vi "GetProperties.vi"(8 "error in":errorcluster, 11 "Numeric in":refnum<class "Numeric.lvclass">) -> (0 "error out":errorcluster, 3 "Numeric out":refnum<class "Numeric.lvclass">)   [LabVIEW 2014, in "Numeric.lvclass"]
uses:
  Numeric.lvclass
  Numeric.lvclass/Numeric.ctl
  Control/Control.lvclass
  Text/Text.lvclass
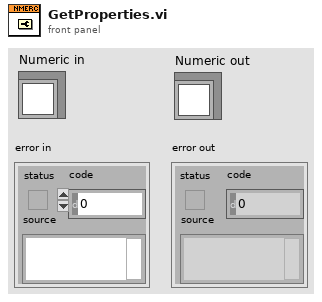
[diagram p1: front panel]
types:
  T1 = typedef "LVMinMaxIncTypeDef.ctl" = cluster{"Minimum":dbl, "Maximum":dbl, "Increment":dbl}
  T2 = typedef "LVKeyTypeDef.ctl" = cluster{"Focus":bool, "Control":bool, "Shift":bool, "Key":string}
  T3 = typedef "LVNumericRepresentation.ctl" = enum32{"Extended Precision", "Double Precision", "Single Precision", "Long", "Word", "Byte", "Unsigned Long", "Unsigned Word", "Unsigned Byte", "Complex Extended", "Complex Double", "Complex Single", "Quad", "Unsigned Quad", "Fixed-Point"}
  T4 = typedef "LVOutOfRangeActionTypeDef.ctl" = cluster{"OutOfRngActMin":u8, "OutOfRngActMax":u8, "OutOfRngActInc":u8}
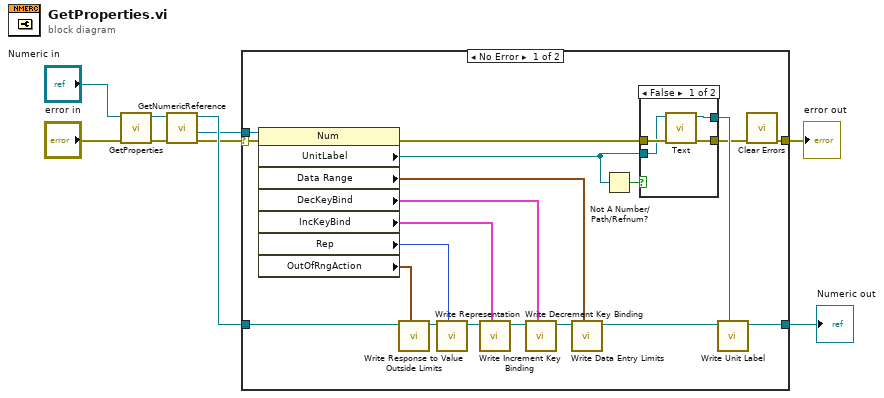
[diagram p0: block diagram]
diagram:
  n1 = call-parent "GetProperties.vi"("error in"="error in", "Control in"="Numeric in") -> ("error out"=w1:errorcluster, "Control out"=w4:refnum<class "Numeric.lvclass">)  [unwired: 8 in]
  n2 = call "GetNumericReference.vi"("error in"=w1, "Numeric in"=w4) -> ("error out"=w6:errorcluster, "Numeric reference"=w5:refnum<vi>, "Numeric out"=w7:refnum<class "Numeric.lvclass">)  [unwired: 7 in]
  n3 = case shown="No Error" w6 {
    selector: w6 -> [w29 w36]
    tunnel: [w10 w36] -> w9
    tunnel: [w12 w35] -> w8
    tunnel: w5 -> [w28 _]
    tunnel: w7 -> [w13 w35]
    frame No Error {
      n4 = property class="Num"(reference=w28, error in=w29) -> (error out=w27:errorcluster, "UnitLabel"=w25:refnum<vi>, "Data Range"=w17:T1, "DecKeyBind"=w18:T2, "IncKeyBind"=w19:T2, "Rep"=w22:T3, "OutOfRngAction"=w23:T4)  [unwired: 1 out]
      n5 = call "Write Response to Value Outside Limits.vi"("Out of Range Action"=w23, "Numeric in"=w13) -> ("Numeric out"=w21:refnum<class "Numeric.lvclass">)  [unwired: 7 in]
      n6 = call "Write Representation.vi"("Numeric Representation"=w22, "Numeric in"=w21) -> ("Numeric out"=w20:refnum<class "Numeric.lvclass">)  [unwired: 7 in]
      n7 = call "Write Increment Key Binding.vi"("Increment Key Binding"=w19, "Numeric in"=w20) -> ("Numeric out"=w16:refnum<class "Numeric.lvclass">)  [unwired: 7 in]
      n8 = call "Write Decrement Key Binding.vi"("Decrement Key Binding"=w18, "Numeric in"=w16) -> ("Numeric out"=w15:refnum<class "Numeric.lvclass">)  [unwired: 7 in]
      n9 = call "Write Data Entry Limits.vi"("Data Entry Limits"=w17, "Numeric in"=w15) -> ("Numeric out"=w14:refnum<class "Numeric.lvclass">)  [unwired: 7 in]
      n10 = Not A Number/Path/Refnum?(number/path/refnum=w25) -> (NaN/Path/Refnum?=w26:bool)
      n11 = case shown="False" w26 {
        tunnel: w27 -> [w33 w34]
        tunnel: w25 -> [w32 _]
        tunnel: [w31 _] -> w24
        tunnel: [w30 w34] -> w11
        frame False {
          n12 = call "Text.vi"("error in"=w33, "Gen Refnum"=w32) -> ("error out"=w30:errorcluster, "Text out"=w31:refnum<class "Text.lvclass">)  [unwired: 8 in]
        }
        frame True {
        }
      }
      n13 = call "Write Unit Label.vi"("Unit Label"=w24, "Numeric in"=w14) -> ("Numeric out"=w12:refnum<class "Numeric.lvclass">)  [unwired: 7 in]
      n14 = call <vilib>:"Clear Errors.vi"("error in (no error)"=w11) -> ("error out"=w10:errorcluster)  [unwired: 5 in, 1 out]
    }
    frame Error {
    }
  }
  "error out" <- w9
  "Numeric out" <- w8
